vi "4-2 matrice 3xM.vi"(0 "Numero di colonne":i32) -> (1 "vettore terza riga":dbl[](array[numeric]) format="%.2f", 2 "Matrice":dbl[][](array[numeric]) format="%.2f")   [LabVIEW 2012]
panel:
  # "Questo programma genera una matrice casuale 3xN con N impostato da pannello"
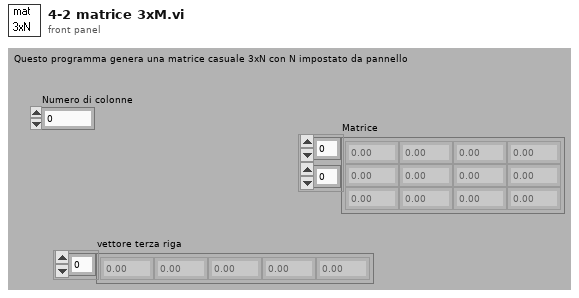
[diagram p1: front panel]
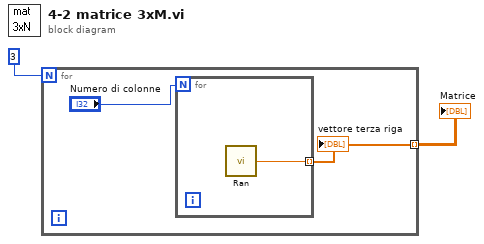
[diagram p0: block diagram]
diagram:
  n1 = for {
    N: 3 ("Numero di colonne") -> [_]
    tunnel: [w3] -> w1 mode=indexing
    n2 = for {
      N: "Numero di colonne" -> [_]
      tunnel: [w5] -> w3 mode=indexing
      n3 = call "Ran.vi"() -> ("out num"=w5:dbl)  [unwired: 5 in]
    }
    "vettore terza riga" <- w3
  }
  "Matrice" <- w1
